vi "Read.vi"(8 "error in (no error)":errorcluster, 10 "delta connection? (F)":bool, 11 "number of modules":i16) -> (0 "error out":errorcluster, 2 "Data Array":sgl[](array[numeric]) format="%.2f")   [LabVIEW 2017, in "MCSA_API.lvlib"]
uses:
  <vilib>/addons/InsightCM/Devices/Shared/Mcsa/Fpga/McsaAcquire/subVIs/McsaAPI/MCSA_API.lvlib
  <vilib>/eio/EIONode/EIONode.xnode
  <vilib>/rvi/eio/common/nirviEmuTemplateMethod_errors.vi
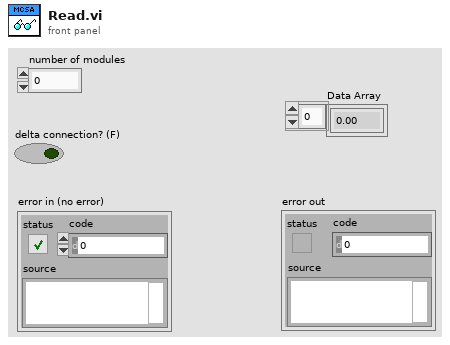
[diagram p1: front panel]
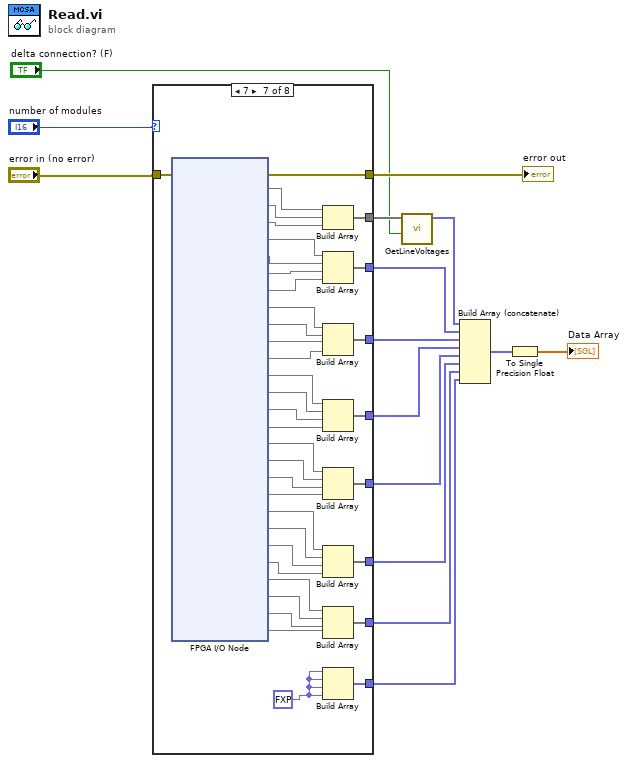
[diagram p0: block diagram]
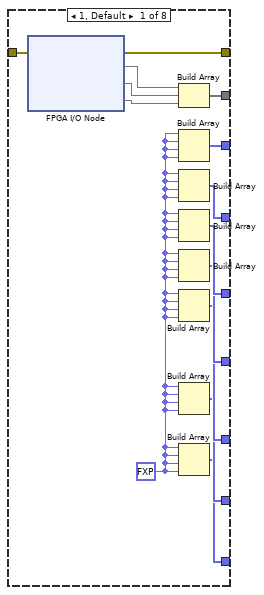
[diagram p2: hidden frame]
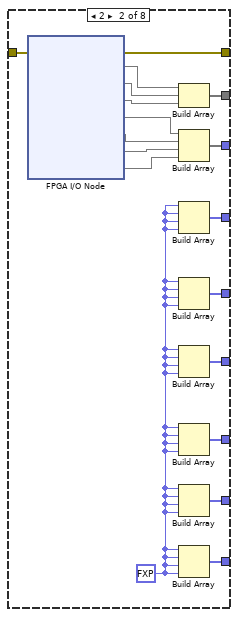
[diagram p3: hidden frame]
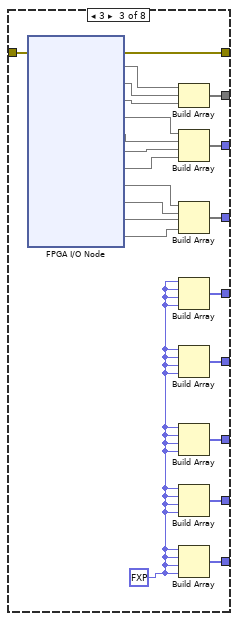
[diagram p4: hidden frame]
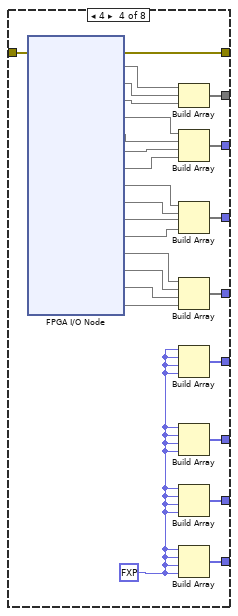
[diagram p5: hidden frame]
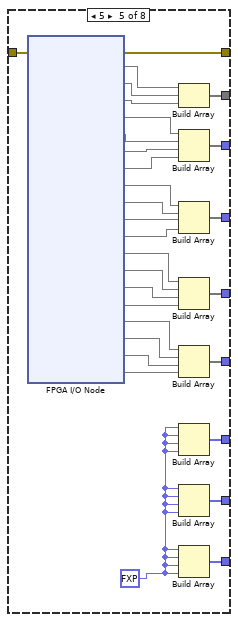
[diagram p6: hidden frame]
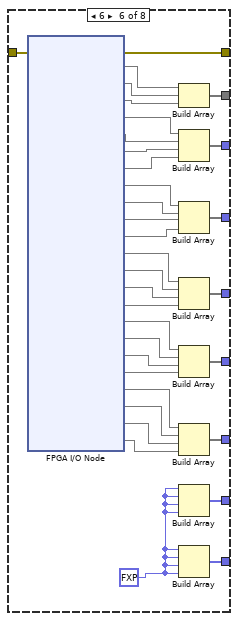
[diagram p7: hidden frame]
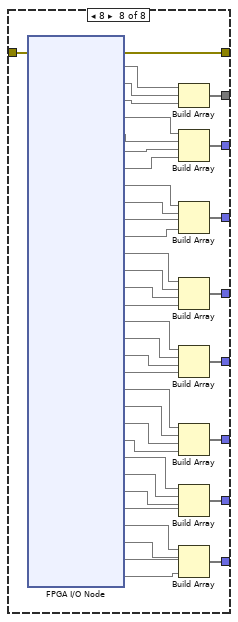
[diagram p8: hidden frame]
diagram:
  n1 = case shown="7" "number of modules" {
    tunnel: "error in (no error)" -> [w26 w44 w66 w92 w122 w156 w194 w235]
    tunnel: [w25 w43 w65 w91 w121 w155 w193 w234] -> w15
    tunnel: [w24 w42 w64 w90 w120 w154 w192 w233] -> w3
    tunnel: [w23 w30 w53 w79 w109 w143 w181 w222] -> w14
    tunnel: [w22 w41 w63 w89 w119 w153 w191 w232] -> w13
    tunnel: [w21 w40 w62 w88 w118 w152 w190 w231] -> w12
    tunnel: [w20 w39 w61 w87 w117 w151 w189 w230] -> w11
    tunnel: [w19 w38 w60 w86 w116 w150 w188 w229] -> w10
    tunnel: [w18 w37 w59 w85 w115 w149 w187 w228] -> w9
    tunnel: [w17 w36 w58 w84 w114 w148 w186 w227] -> w8
    frame 1, Default {
      w16 = fxp<+/-,24,7> 0.0 ("Mod1/AI2")
      n2 = xnode "FPGA I/O Node"("error in"=w26) -> ("error out"=w25:errorcluster, "Mod1/AI0"=w27, "Mod1/AI1"=w29, "Mod1/AI2"=w28)  [unwired: 3 in, 3 out]
      n3 = Build Array(w27, w29, w28) -> (w24:void[])
      n4 = Build Array(w16, w16, w16, w16) -> (w23:fxp<+/-,24,7>[])
      n5 = Build Array(w16, w16, w16, w16) -> (w22:fxp<+/-,24,7>[])
      n6 = Build Array(w16, w16, w16, w16) -> (w21:fxp<+/-,24,7>[])
      n7 = Build Array(w16, w16, w16, w16) -> (w20:fxp<+/-,24,7>[])
      n8 = Build Array(w16, w16, w16, w16) -> (w19:fxp<+/-,24,7>[])
      n9 = Build Array(w16, w16, w16, w16) -> (w18:fxp<+/-,24,7>[])
      n10 = Build Array(w16, w16, w16, w16) -> (w17:fxp<+/-,24,7>[])
    }
    frame 2 {
      w35 = fxp<+/-,24,5> 0.0 ("Mod1/AI2")
      n11 = xnode "FPGA I/O Node"("error in"=w44) -> ("error out"=w43:errorcluster, "Mod1/AI0"=w45, "Mod1/AI1"=w47, "Mod1/AI2"=w46, "Mod2/AI0"=w34, "Mod2/AI1"=w33, "Mod2/AI2"=w32, "Mod2/AI3"=w31)  [unwired: 7 in, 7 out]
      n12 = Build Array(w45, w47, w46) -> (w42:void[])
      n13 = Build Array(w34, w33, w32, w31) -> (w30:void[])
      n14 = Build Array(w35, w35, w35, w35) -> (w41:fxp<+/-,24,5>[])
      n15 = Build Array(w35, w35, w35, w35) -> (w40:fxp<+/-,24,5>[])
      n16 = Build Array(w35, w35, w35, w35) -> (w39:fxp<+/-,24,5>[])
      n17 = Build Array(w35, w35, w35, w35) -> (w38:fxp<+/-,24,5>[])
      n18 = Build Array(w35, w35, w35, w35) -> (w37:fxp<+/-,24,5>[])
      n19 = Build Array(w35, w35, w35, w35) -> (w36:fxp<+/-,24,5>[])
    }
    frame 3 {
      w48 = fxp<+/-,24,5> 0.0 ("Mod1/AI2")
      n20 = xnode "FPGA I/O Node"("error in"=w66) -> ("error out"=w65:errorcluster, "Mod1/AI0"=w67, "Mod1/AI1"=w69, "Mod1/AI2"=w68, "Mod2/AI0"=w57, "Mod2/AI1"=w56, "Mod2/AI2"=w55, "Mod2/AI3"=w54, "Mod3/AI0"=w52, "Mod3/AI1"=w51, "Mod3/AI2"=w50, "Mod3/AI3"=w49)  [unwired: 11 in, 11 out]
      n21 = Build Array(w67, w69, w68) -> (w64:void[])
      n22 = Build Array(w57, w56, w55, w54) -> (w53:void[])
      n23 = Build Array(w52, w51, w50, w49) -> (w63:void[])
      n24 = Build Array(w48, w48, w48, w48) -> (w62:fxp<+/-,24,5>[])
      n25 = Build Array(w48, w48, w48, w48) -> (w61:fxp<+/-,24,5>[])
      n26 = Build Array(w48, w48, w48, w48) -> (w60:fxp<+/-,24,5>[])
      n27 = Build Array(w48, w48, w48, w48) -> (w59:fxp<+/-,24,5>[])
      n28 = Build Array(w48, w48, w48, w48) -> (w58:fxp<+/-,24,5>[])
    }
    frame 4 {
      w70 = fxp<+/-,24,5> 0.0 ("Mod1/AI2")
      n29 = xnode "FPGA I/O Node"("error in"=w92) -> ("error out"=w91:errorcluster, "Mod1/AI0"=w93, "Mod1/AI1"=w95, "Mod1/AI2"=w94, "Mod2/AI0"=w83, "Mod2/AI1"=w82, "Mod2/AI2"=w81, "Mod2/AI3"=w80, "Mod3/AI0"=w78, "Mod3/AI1"=w77, "Mod3/AI2"=w76, "Mod3/AI3"=w75, "Mod4/AI0"=w74, "Mod4/AI1"=w73, "Mod4/AI2"=w72, "Mod4/AI3"=w71)  [unwired: 15 in, 15 out]
      n30 = Build Array(w93, w95, w94) -> (w90:void[])
      n31 = Build Array(w83, w82, w81, w80) -> (w79:void[])
      n32 = Build Array(w78, w77, w76, w75) -> (w89:void[])
      n33 = Build Array(w74, w73, w72, w71) -> (w88:void[])
      n34 = Build Array(w70, w70, w70, w70) -> (w87:fxp<+/-,24,5>[])
      n35 = Build Array(w70, w70, w70, w70) -> (w86:fxp<+/-,24,5>[])
      n36 = Build Array(w70, w70, w70, w70) -> (w85:fxp<+/-,24,5>[])
      n37 = Build Array(w70, w70, w70, w70) -> (w84:fxp<+/-,24,5>[])
    }
    frame 5 {
      w96 = fxp<+/-,24,5> 0.0 ("Mod1/AI2")
      n38 = xnode "FPGA I/O Node"("error in"=w122) -> ("error out"=w121:errorcluster, "Mod1/AI0"=w123, "Mod1/AI1"=w125, "Mod1/AI2"=w124, "Mod2/AI0"=w113, "Mod2/AI1"=w112, "Mod2/AI2"=w111, "Mod2/AI3"=w110, "Mod3/AI0"=w108, "Mod3/AI1"=w107, "Mod3/AI2"=w106, "Mod3/AI3"=w105, "Mod4/AI0"=w104, "Mod4/AI1"=w103, "Mod4/AI2"=w102, "Mod4/AI3"=w101, "Mod5/AI0"=w100, "Mod5/AI1"=w99, "Mod5/AI2"=w98, "Mod5/AI3"=w97)  [unwired: 19 in, 19 out]
      n39 = Build Array(w123, w125, w124) -> (w120:void[])
      n40 = Build Array(w113, w112, w111, w110) -> (w109:void[])
      n41 = Build Array(w108, w107, w106, w105) -> (w119:void[])
      n42 = Build Array(w104, w103, w102, w101) -> (w118:void[])
      n43 = Build Array(w100, w99, w98, w97) -> (w117:void[])
      n44 = Build Array(w96, w96, w96, w96) -> (w116:fxp<+/-,24,5>[])
      n45 = Build Array(w96, w96, w96, w96) -> (w115:fxp<+/-,24,5>[])
      n46 = Build Array(w96, w96, w96, w96) -> (w114:fxp<+/-,24,5>[])
    }
    frame 6 {
      w126 = fxp<+/-,24,5> 0.0 ("Mod1/AI2")
      n47 = xnode "FPGA I/O Node"("error in"=w156) -> ("error out"=w155:errorcluster, "Mod1/AI0"=w157, "Mod1/AI1"=w159, "Mod1/AI2"=w158, "Mod2/AI0"=w147, "Mod2/AI1"=w146, "Mod2/AI2"=w145, "Mod2/AI3"=w144, "Mod3/AI0"=w142, "Mod3/AI1"=w141, "Mod3/AI2"=w140, "Mod3/AI3"=w139, "Mod4/AI0"=w138, "Mod4/AI1"=w137, "Mod4/AI2"=w136, "Mod4/AI3"=w135, "Mod5/AI0"=w134, "Mod5/AI1"=w133, "Mod5/AI2"=w132, "Mod5/AI3"=w131, "Mod6/AI0"=w130, "Mod6/AI1"=w129, "Mod6/AI2"=w128, "Mod6/AI3"=w127)  [unwired: 23 in, 23 out]
      n48 = Build Array(w157, w159, w158) -> (w154:void[])
      n49 = Build Array(w147, w146, w145, w144) -> (w143:void[])
      n50 = Build Array(w142, w141, w140, w139) -> (w153:void[])
      n51 = Build Array(w138, w137, w136, w135) -> (w152:void[])
      n52 = Build Array(w134, w133, w132, w131) -> (w151:void[])
      n53 = Build Array(w130, w129, w128, w127) -> (w150:void[])
      n54 = Build Array(w126, w126, w126, w126) -> (w149:fxp<+/-,24,5>[])
      n55 = Build Array(w126, w126, w126, w126) -> (w148:fxp<+/-,24,5>[])
    }
    frame 7 {
      w160 = fxp<+/-,24,5> 0.0 ("Mod1/AI2")
      n56 = xnode "FPGA I/O Node"("error in"=w194) -> ("error out"=w193:errorcluster, "Mod1/AI0"=w195, "Mod1/AI1"=w197, "Mod1/AI2"=w196, "Mod2/AI0"=w185, "Mod2/AI1"=w184, "Mod2/AI2"=w183, "Mod2/AI3"=w182, "Mod3/AI0"=w180, "Mod3/AI1"=w179, "Mod3/AI2"=w178, "Mod3/AI3"=w177, "Mod4/AI0"=w176, "Mod4/AI1"=w175, "Mod4/AI2"=w174, "Mod4/AI3"=w173, "Mod5/AI0"=w172, "Mod5/AI1"=w171, "Mod5/AI2"=w170, "Mod5/AI3"=w169, "Mod6/AI0"=w168, "Mod6/AI1"=w167, "Mod6/AI2"=w166, "Mod6/AI3"=w165, "Mod7/AI0"=w164, "Mod7/AI1"=w163, "Mod7/AI2"=w162, "Mod7/AI3"=w161)  [unwired: 27 in, 27 out]
      n57 = Build Array(w195, w197, w196) -> (w192:void[])
      n58 = Build Array(w185, w184, w183, w182) -> (w181:void[])
      n59 = Build Array(w180, w179, w178, w177) -> (w191:void[])
      n60 = Build Array(w176, w175, w174, w173) -> (w190:void[])
      n61 = Build Array(w172, w171, w170, w169) -> (w189:void[])
      n62 = Build Array(w168, w167, w166, w165) -> (w188:void[])
      n63 = Build Array(w164, w163, w162, w161) -> (w187:void[])
      n64 = Build Array(w160, w160, w160, w160) -> (w186:fxp<+/-,24,5>[])
    }
    frame 8 {
      n65 = xnode "FPGA I/O Node"("error in"=w235) -> ("error out"=w234:errorcluster, "Mod1/AI0"=w236, "Mod1/AI1"=w238, "Mod1/AI2"=w237, "Mod2/AI0"=w226, "Mod2/AI1"=w225, "Mod2/AI2"=w224, "Mod2/AI3"=w223, "Mod3/AI0"=w221, "Mod3/AI1"=w220, "Mod3/AI2"=w219, "Mod3/AI3"=w218, "Mod4/AI0"=w217, "Mod4/AI1"=w216, "Mod4/AI2"=w215, "Mod4/AI3"=w214, "Mod5/AI0"=w213, "Mod5/AI1"=w212, "Mod5/AI2"=w211, "Mod5/AI3"=w210, "Mod6/AI0"=w209, "Mod6/AI1"=w208, "Mod6/AI2"=w207, "Mod6/AI3"=w206, "Mod7/AI0"=w205, "Mod7/AI1"=w204, "Mod7/AI2"=w203, "Mod7/AI3"=w202, "Mod8/AI0"=w201, "Mod8/AI1"=w200, "Mod8/AI2"=w199, "Mod8/AI3"=w198)  [unwired: 31 in, 31 out]
      n66 = Build Array(w236, w238, w237) -> (w233:void[])
      n67 = Build Array(w226, w225, w224, w223) -> (w222:void[])
      n68 = Build Array(w221, w220, w219, w218) -> (w232:void[])
      n69 = Build Array(w217, w216, w215, w214) -> (w231:void[])
      n70 = Build Array(w213, w212, w211, w210) -> (w230:void[])
      n71 = Build Array(w209, w208, w207, w206) -> (w229:void[])
      n72 = Build Array(w205, w204, w203, w202) -> (w228:void[])
      n73 = Build Array(w201, w200, w199, w198) -> (w227:void[])
    }
  }
  "error out" <- w15
  n74 = call <vilib>:"GetLineVoltages.vi"("delta connection? (F)"="delta connection? (F)", "original voltages"=w3) -> ("line or phase voltages"=w2:fxp<+/-,25,11>[])  [unwired: 9 in]
  n75 = Build Array (concatenate)(w2, w14, w13, w12, w11, w10, w9, w8) -> (w7:fxp<+/-,30,11>[])
  n76 = To Single Precision Float(number=w7) -> (single precision float=→"Data Array":sgl[])
